vi "Set field.vi"(2 "Calibration parameters":T1={"Electromagnet Calibration (mT/Volt)"=-234.77, "Set field (mT)"=0}, 3 "Channel parameters":T2={"Com port"="GPIB0::9::INSTR", "DAC channel"=1} {"DAC channel" min=1 max=4 step=1}) -> ()   [LabVIEW 2018]
panel:
  in  "error in (no error)":errorcluster
  out "error out":errorcluster
  in  "millisecond timer value":u32
  # "use if 0 V programming voltage\nresults in a finite offset current."
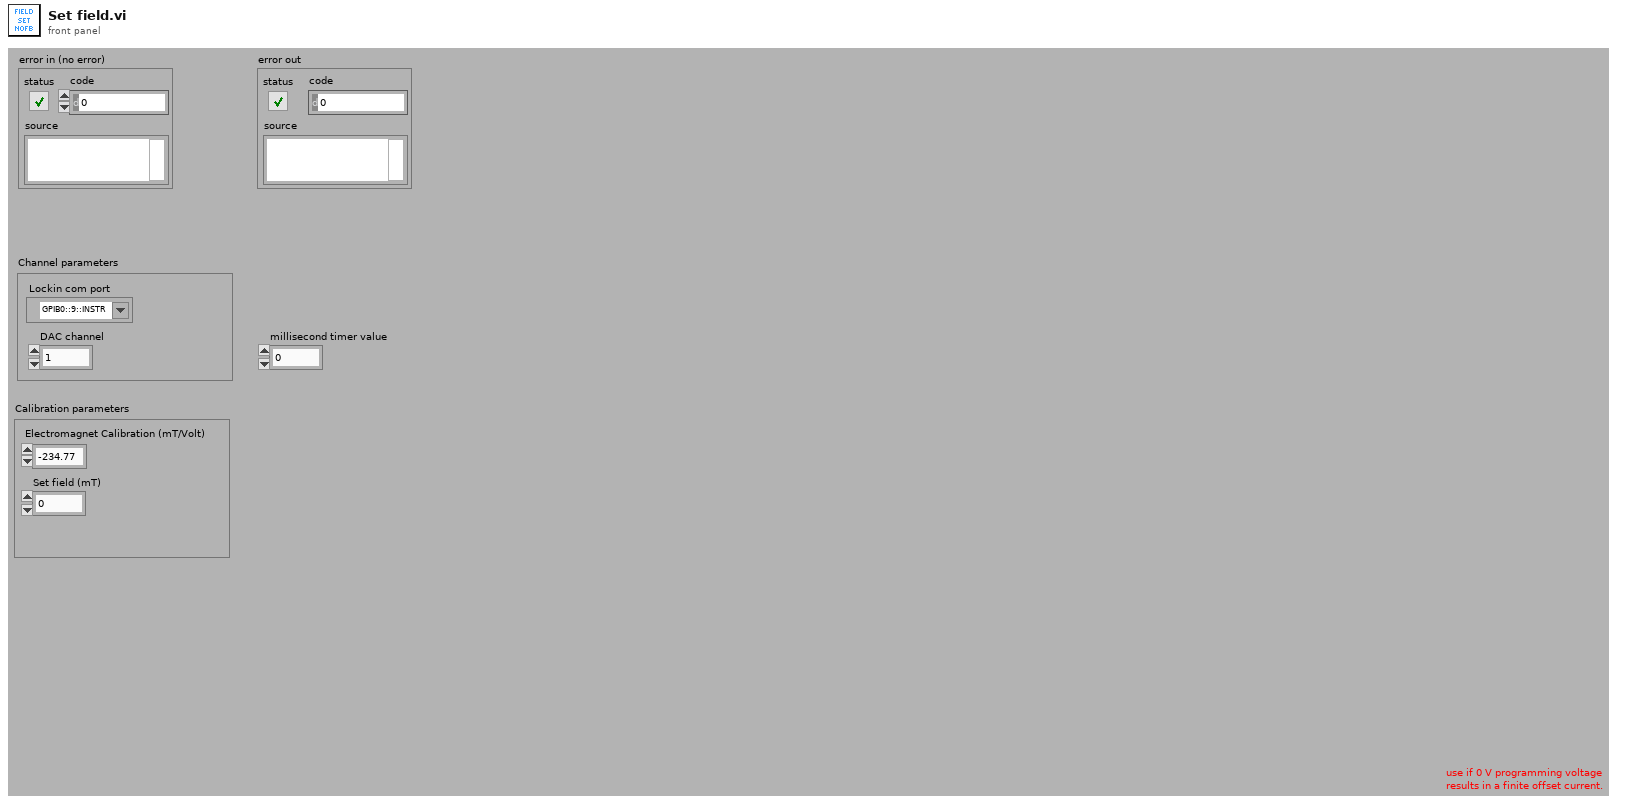
[diagram p1: front panel]
types:
  T1 = cluster{"Electromagnet Calibration (mT/Volt)":dbl, "Set field (mT)":i32}
  T2 = cluster{"Com port":refnum<visa-resource-name>, "DAC channel":u16}
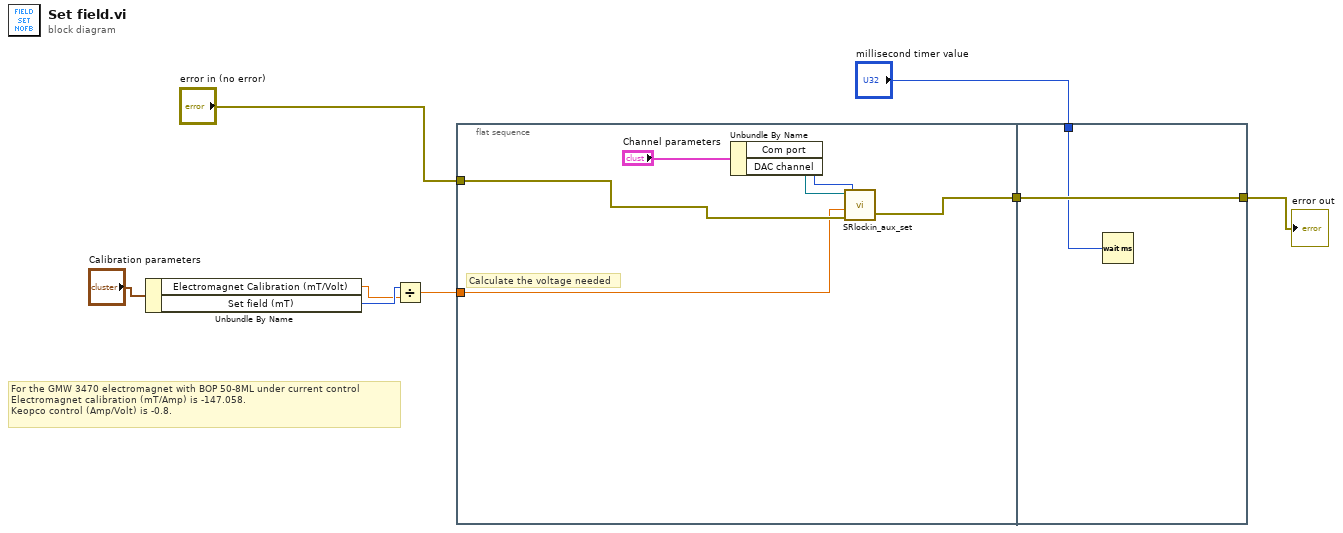
[diagram p0: block diagram]
diagram:
  # "For the GMW 3470 electromagnet with BOP 50-8ML under current control\nElectromagnet calibration (mT/Amp) is -147.058.\nKeopco control (Amp/Volt) is -0.8."
  n1 = Unbundle By Name("Calibration parameters") -> ("Electromagnet Calibration (mT/Volt)"=w1:dbl, "Set field (mT)"=w2:i32)
  n2 = Divide(x=w2, y=w1) -> (x/y=w3:dbl)
  n3 = flat-sequence {
    tunnel: [w14] -> w7
    tunnel: "error in (no error)" -> [w10]
    tunnel: w3 -> [w9]
    tunnel: [w16] -> w5
    tunnel: w7 -> [w16]
    tunnel: "millisecond timer value" -> [w15]
    frame #0 {
      # "Calculate the voltage needed"
      n4 = Unbundle By Name("Channel parameters") -> ("Com port"=w12:refnum<visa-resource-name>, "DAC channel"=w11:u16)
      n5 = call "SRlockin_aux_set.vi"("error in (no error)"=w10, "Set Voltage (V)"=w9, "DAC channel"=w11, "VISA resource name"=w12) -> ("error out"=w14:errorcluster)  [unwired: 1 out]
    }
    frame #1 {
      n6 = Wait (ms)(milliseconds to wait=w15) -> ()  [unwired: 1 out]
    }
  }
  "error out" <- w5
